vi "setAO_DC.vi"(8 "error in (no error)":errorcluster, 9 "DC (V)":dbl, 10 "AO Channel":T1=1 min=1 max=16, 11 "Instrument.Lockin in":refnum<class "Instrument.Lockin.lvclass">) -> (0 "error out":errorcluster, 3 "Instrument.Lockin out":refnum<class "Instrument.Lockin.lvclass">)   [LabVIEW 2016, in "Instrument.Lockin.lvclass"]
doc: "API to configure an AO DC offset.\n\nSpecify which channel you want to change and the value you want to set.\n\nIf address=\"\", this API reads from localhost\nIf address is remote lockin, you need to add this computer to allowed whitelist on the lockin computer you are trying to access."
uses:
  Instrument.Lockin.lvclass
  LockinDAQ/Typedefs/AO_Channel-Numeric.ctl
  Typedefs/Instrument.Lockin.Commands--Enum.ctl
  LockinDAQ/LockinDAQ.lvclass
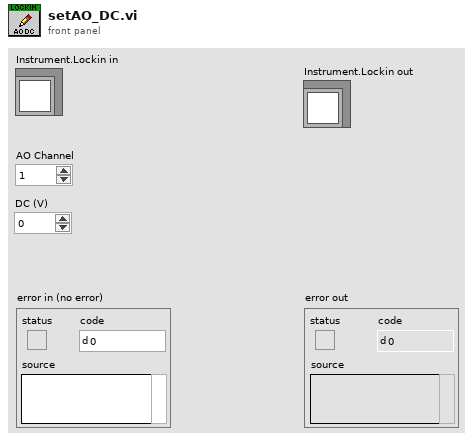
[diagram p1: front panel]
types:
  T1 = typedef "LockinDAQ.lvclass/AO_Channel-Numeric.ctl" = i32
  T2 = typedef "Instrument.Lockin.lvclass/Instrument.Lockin.Commands--Enum.ctl" = enum16{"setAO", "setAO_Amplitude", "setAO_DC", "setAO_Frequency", "setAO_Phase", "setAO_Function", "setAO_I+", "setREF", "setREF_Frequency", "setREF_Phase", "setIVmode", "Reset", "setSampling", "Trigger", "getAO", "getAI", "getResults", "getTrigger", "getIVmode", "getSampling", "getAOconfig", "getREFconfig", "setGain", "getGain", "setAutoSampling", "getAutoSampling", "setSweep", "getStatus", "getSweepResults", "getIVSweepResults", "startSweep", "stopSweep", "setAUX", "getAUX"}
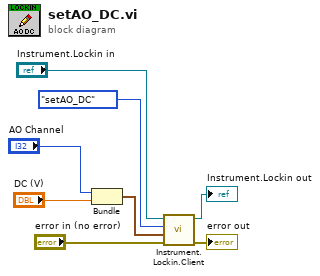
[diagram p0: block diagram]
diagram:
  n1 = Bundle("AO Channel"="AO Channel", "DC (V)"="DC (V)") -> (w8:cluster{"AO Channel":T1, "DC (V)":dbl})  [unwired: 1 in]
  n2 = call "Instrument.Lockin.Client.vi"("error in (no error)"="error in (no error)", "Data"=w8, "Command"=Instrument.Lockin.Commands--Enum."setAO_DC", "Instrument.Lockin in"="Instrument.Lockin in") -> ("error out"=→"error out":errorcluster, "Instrument.Lockin out"=→"Instrument.Lockin out":refnum<class "Instrument.Lockin.lvclass">)  [unwired: 5 in, 1 out]
